vi "Get Ancestors.vi"(5 "Exclude Self (T)":bool=TRUE, 7 "Exclude LabVIEW Object (T)":bool=TRUE, 8 "error in (no error)":errorcluster, 11 "LabVIEW Object":refnum<class>) -> (0 "error out":errorcluster, 2 "Ancestor Class Names":string[](array[string]), 3 "Ancestors":refnum<class>[](array[class]))   [LabVIEW 2017, in "Composition.lvlib"]
uses:
  Composition.lvlib
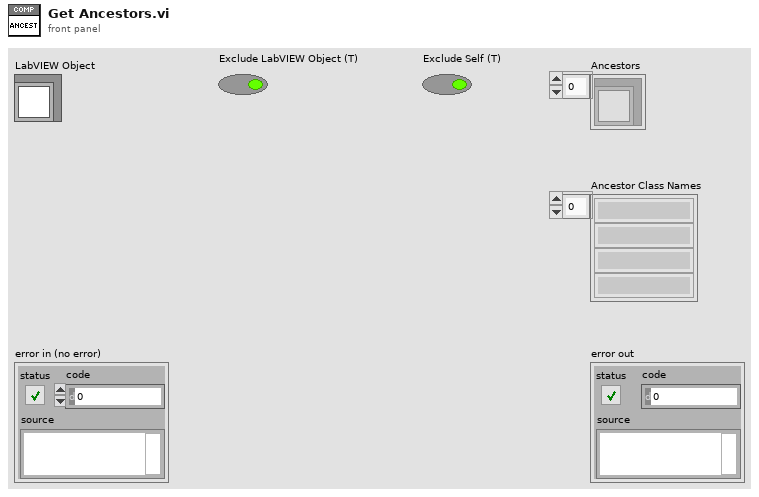
[diagram p1: front panel]
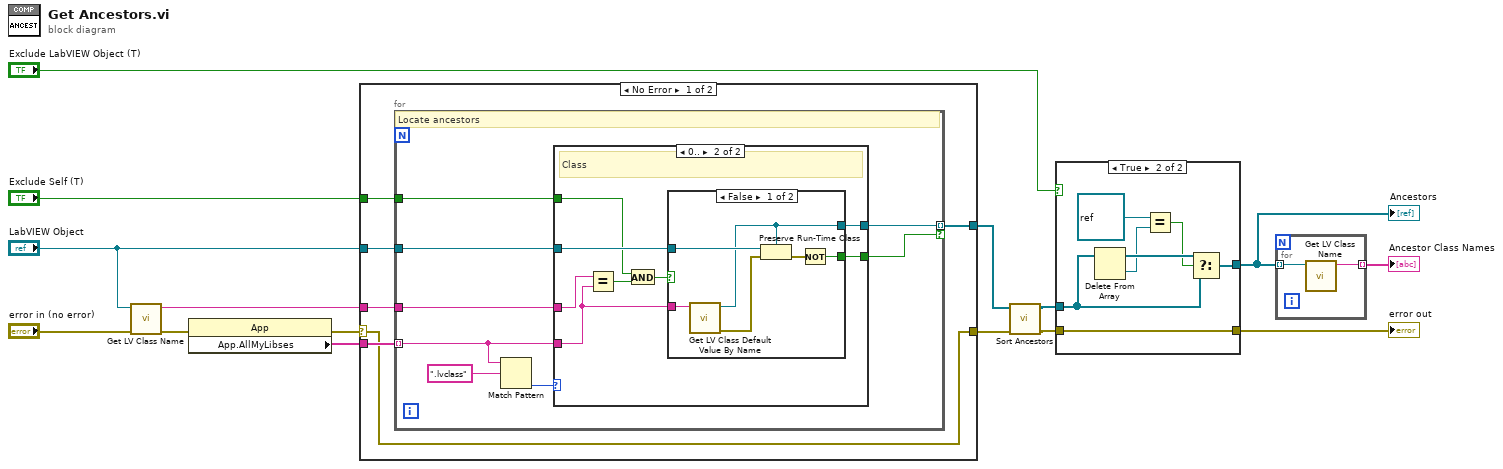
[diagram p0: block diagram]
diagram:
  n1 = call <vilib>:"Get LV Class Name.vi"("error in (no error)"="error in (no error)", "object"="LabVIEW Object") -> ("error out"=w11:errorcluster, "class name"=w14:string)  [unwired: 8 in]
  n2 = property class="App"(error in=w11) -> (error out=w2:errorcluster, "App.AllMyLibses"=w13:string[])  [unwired: 1 in, 1 out]
  n3 = case shown="No Error" w2 {
    selector: w2 -> [w16 w44]
    tunnel: w14 -> [w21 _]
    tunnel: w13 -> [w20 _]
    tunnel: "LabVIEW Object" -> [w19 _]
    tunnel: [w18 _] -> w9
    tunnel: "Exclude Self (T)" -> [w17 _]
    tunnel: [w16 w44] -> w1
    frame No Error {
      n4 = for {
        tunnel: w20 -> [w29] mode=indexing
        tunnel: [w26] -> w18 mode=indexing if=w25
        tunnel: w19 -> [w24]
        tunnel: w21 -> [w23]
        tunnel: w17 -> [w22]
        # "Locate ancestors"
        n5 = Match Pattern(string=w29, regular expression=".lvclass") -> (offset past match=w28:i32)  [unwired: 1 in, 3 out]
        n6 = case shown="0.." w28 {
          tunnel: [_ w33] -> w26
          tunnel: w29 -> [_ w34]
          tunnel: [_ w37] -> w25
          tunnel: w24 -> [_ w36]
          tunnel: w23 -> [_ w35]
          tunnel: w22 -> [_ w30]
          frame Default {
            # "Not a class"
          }
          frame 0.. {
            # "Class"
            n7 = Equal?(x=w35, y=w34) -> (x = y?=w32:bool)
            n8 = And(x=w30, y=w32) -> (x .and. y?=w31:bool)
            n9 = case shown="False" w31 {
              tunnel: [w43 _] -> w37
              tunnel: w36 -> [w42 _]
              tunnel: w34 -> [w41 _]
              tunnel: [w39 _] -> w33
              frame False {
                n10 = call <vilib>:"Get LV Class Default Value By Name.vi"("class name"=w41) -> ("error out"=w38:errorcluster, "object"=w39:refnum<class>)  [unwired: 9 in]
                n11 = Preserve Run-Time Class(object in=w42, error in=w38, 2:w39) -> (error out=w40:errorcluster)  [unwired: 1 out]
                n12 = Not(x=w40) -> (.not. x?=w43:bool)
              }
              frame True {
              }
            }
          }
        }
      }
    }
    frame Error {
    }
  }
  n13 = call "Sort Ancestors.vi"("error in (no error)"=w1, "Classes"=w9) -> ("error out"=w5:errorcluster, "Sorted Classes"=w8:refnum<class>[])  [unwired: 8 in]
  n14 = case shown="True" "Exclude LabVIEW Object (T)" {
    tunnel: w8 -> [w46 w52]
    tunnel: [w46 w48] -> w7
    tunnel: [w45 w47] -> w6
    tunnel: w5 -> [w45 w47]
    frame False {
    }
    frame True {
      n15 = Delete From Array(array=w52) -> (deleted portion=w50:refnum<class>, array with subset deleted=w53:refnum<class>[])  [unwired: 2 in]
      n16 = Equal?(x=refnum<class> refnum ("object"), y=w50) -> (x = y?=w51:bool)
      n17 = Select(t=w53, s=w51, f=w52) -> (s? t:f=w48:refnum<class>[])
    }
  }
  "Ancestors" <- w7
  "error out" <- w6
  n18 = for {
    tunnel: w7 -> [w55] mode=indexing
    tunnel: [w54] -> w15 mode=indexing
    n19 = call <vilib>:"Get LV Class Name.vi"("object"=w55) -> ("class name"=w54:string)  [unwired: 9 in, 1 out]
  }
  "Ancestor Class Names" <- w15
